vi "toplevel.vi"() -> ()   [LabVIEW 2013]
uses:
  SensorDataType.ctl
panel:
  out "Einfallswinkel":dbl(knob) scale=-90.0..90.0
  out "Sensordaten (Raw)":u16[](graph)
  in  "Simulated Orientation":i8(knob) scale=-90.0..90.0
  out "Simulation":bool
  out "Live-Daten":bool
  in  "Modus Operandi":bool
  out "Sensordaten (Normalisiert)":dbl[](graph)=[0.10526315789473684, 0.15789473684210525, 0.15789473684210525, 0.15789473684210525, 0.15789473684210525, 0.10526315789473684, 0.15789473684210525]
  in  "stop":bool
  in  "Serial Input":refnum<visa-resource-name>="COM6"
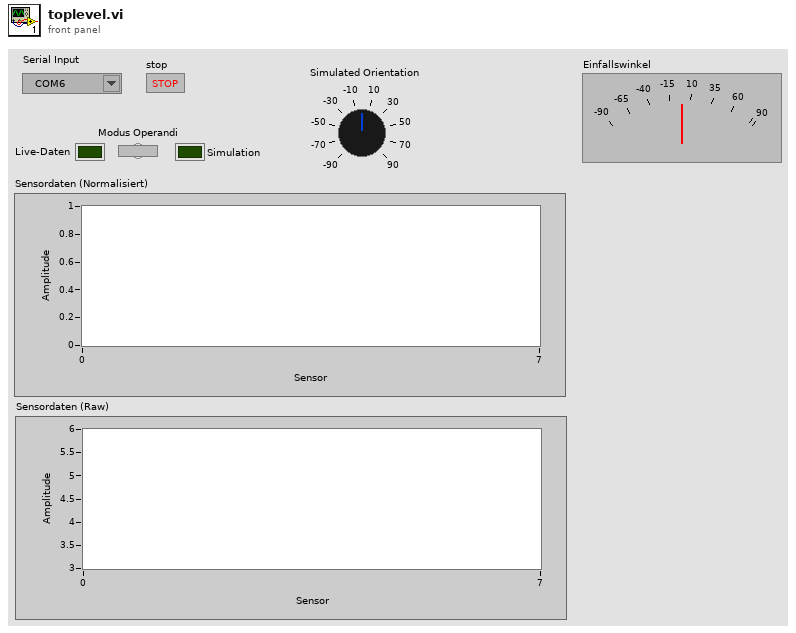
[diagram p1: front panel]
types:
  T1 = enum8{"Enabled", "Disabled", "Disabled and Grayed Out"}
  T2 = typedef "SensorDataType.ctl" = cluster{"Raw":u16[], "Normalized\n":dbl[]}
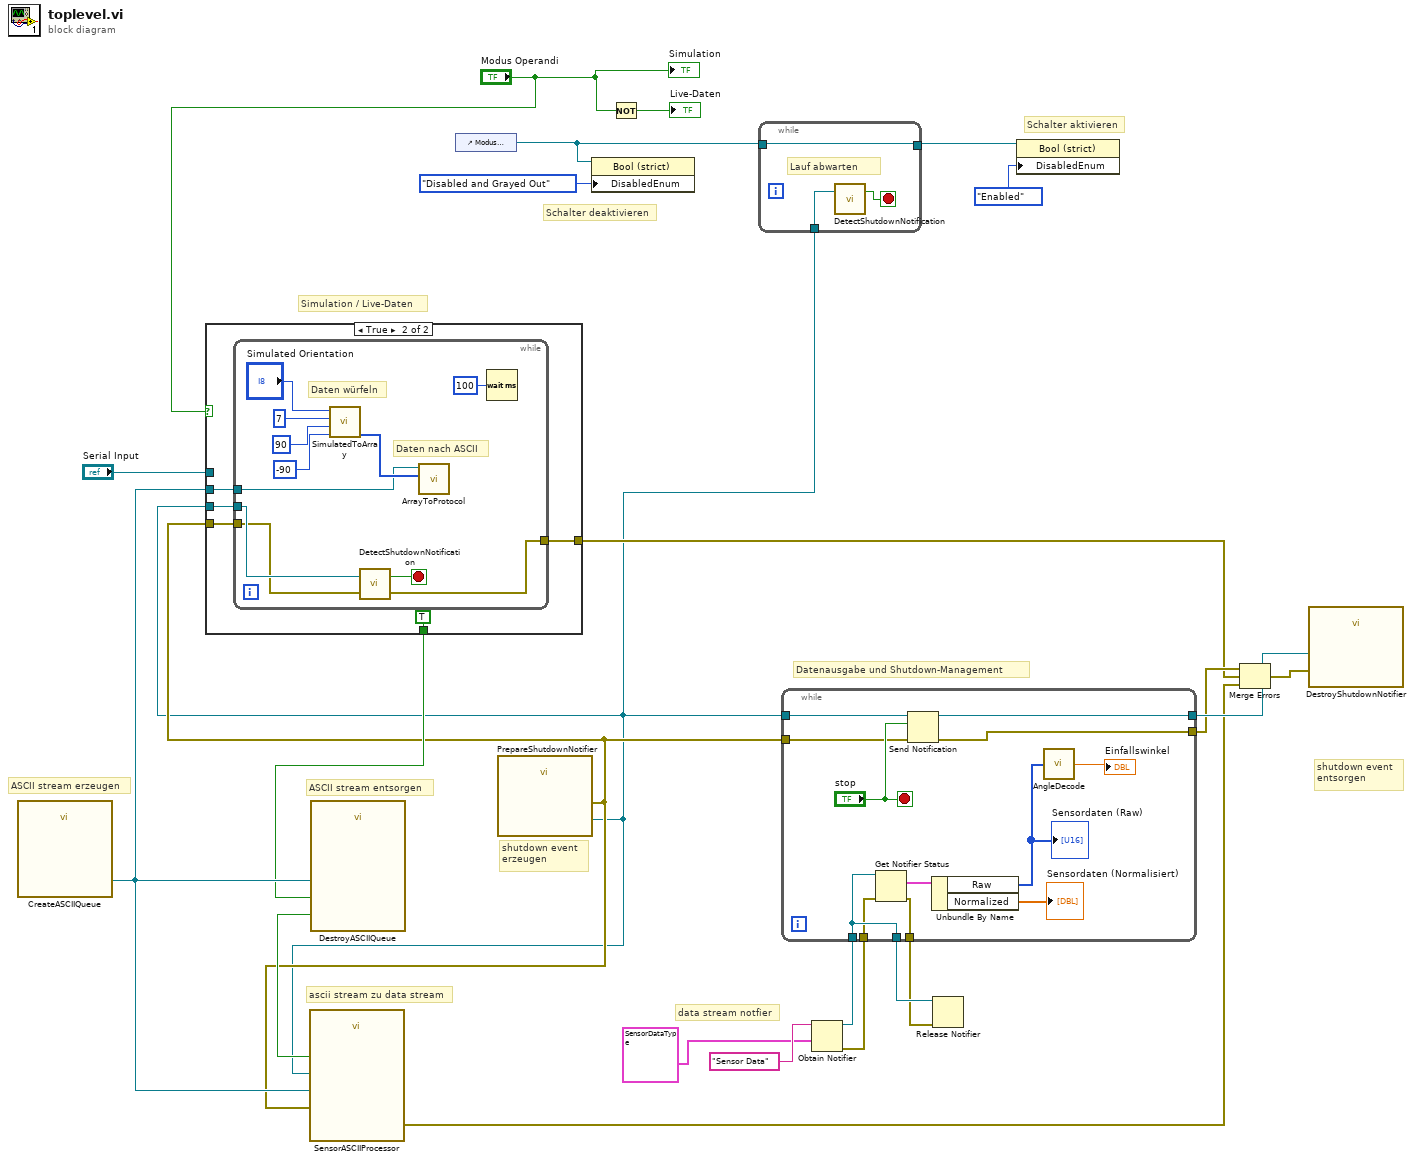
[diagram p0: block diagram]
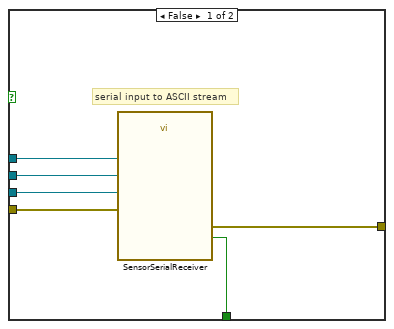
[diagram p2: hidden frame]
diagram:
  # "Simulation / Live-Daten"
  # "Schalter deaktivieren"
  # "Schalter aktivieren"
  # "Datenausgabe und Shutdown-Management"
  # "shutdown event\nentsorgen"
  # "data stream notfier"
  # "shutdown event\nerzeugen"
  # "ASCII stream entsorgen"
  # "ASCII stream erzeugen"
  # "ascii stream zu data stream"
  n1 = call "CreateASCIIQueue.vi"() -> ("Queue out"=w20:refnum<queue>)  [unwired: 11 in]
  n2 = control-ref of="Modus Operandi"() -> (w3:refnum<vi>)
  n3 = call "PrepareShutdownNotifier.vi"() -> ("error out"=w8:errorcluster, "Notifier out"=w7:refnum<notifier>)  [unwired: 10 in]
  n4 = case shown="True" "Modus Operandi" {
    tunnel: "Serial Input" -> [w29 _]
    tunnel: w20 -> [w28 w30]
    tunnel: [w27 w32] -> w19
    tunnel: [w26 TRUE ("Done")] -> w15
    tunnel: w8 -> [w25 w31]
    tunnel: w7 -> [w24 w34]
    frame False {
      # "serial input to ASCII stream"
      n5 = call "SensorSerialReceiver.vi"("Notifier Error In"=w25, "Notifier"=w24, "Queue"=w28, "VISA resource name"=w29) -> ("Notifier Error Out"=w27:errorcluster, "Done"=w26:bool)  [unwired: 6 in]
    }
    frame True {
      n6 = while {
        tunnel: w34 -> [w40]
        tunnel: [w39] -> w32
        tunnel: w31 -> [w38]
        tunnel: w30 -> [w36]
        stop <- w41 stop-if-true
        # "Daten nach ASCII"
        # "Daten würfeln"
        n7 = call "SimulatedToArray.vi"("Minimum Angle"=i8 -90, "Maximum Angle"=i8 90, "Number of Elements"=u8 7, "Degree"="Simulated Orientation") -> ("Value Array"=w37:u16[])  [unwired: 7 in]
        n8 = call "DetectShutdownNotification.vi"("error in (no error)"=w38, "Shutdown Notifier"=w40) -> ("error out"=w39:errorcluster, "Shutdown"=w41:bool)
        n9 = call "ArrayToProtocol.vi"("Simulated Data"=w37, "Queue"=w36) -> ()  [unwired: 10 in]
        n10 = Wait (ms)(milliseconds to wait=u32 100) -> ()  [unwired: 1 out]
      }
    }
  }
  n11 = call "SensorASCIIProcessor.vi"("Notifier Error In"=w8, "Shutdown Notifier"=w7, "Queue"=w20) -> ("Notifier Error Out"=w18:errorcluster, "Done"=w17:bool)  [unwired: 4 in]
  n12 = call "DestroyASCIIQueue.vi"("Ready 2"=w17, "Ready 1"=w15, "Queue in"=w20) -> ()  [unwired: 9 in]
  n13 = property on="Property Node" class="Bool (strict)"(reference=w3, "DisabledEnum"=T1."Disabled and Grayed Out" ("Disabled")) -> ()  [unwired: 1 in, 2 out]
  n14 = Not(x="Modus Operandi") -> (.not. x?=→"Live-Daten":bool)
  n15 = while {
    tunnel: w7 -> [w48]
    tunnel: [w46] -> w4
    tunnel: w3 -> [w46]
    stop <- w47 stop-if-true
    # "Lauf abwarten"
    n16 = call "DetectShutdownNotification.vi"("Shutdown Notifier"=w48) -> ("Shutdown"=w47:bool)  [unwired: 1 in, 1 out]
  }
  n17 = Obtain Notifier(name (unnamed)="Sensor Data", notification data type=T2 {"Raw"=[22, 22, 26, 24, 24, 26, 26], "Normalized\n"=[0.12941176470588237, 0.12941176470588237, 0.15294117647058825, 0.1411764705882353, 0.1411764705882353, 0.15294117647058825, 0.15294117647058825]} ("Sensor Data Type")) -> (notifier out=w14:refnum<notifier>, error out=w11:errorcluster)  [unwired: 2 in, 1 out]
  n18 = while {
    tunnel: w7 -> [w51]
    tunnel: [w59] -> w23
    tunnel: [w58] -> w22
    tunnel: w8 -> [w57]
    tunnel: w14 -> [w54]
    tunnel: [w54] -> w13
    tunnel: [w53] -> w12
    tunnel: w11 -> [w52]
    stop <- "stop" stop-if-true
    n19 = Get Notifier Status(notifier=w54, error in (no error)=w52) -> (current notification=w56:T2, error out=w53:errorcluster)  [unwired: 3 out]
    n20 = Send Notification(notification="stop", notifier=w51, error in (no error)=w57) -> (notifier out=w59:refnum<notifier>, error out=w58:errorcluster)
    n21 = Unbundle By Name(w56) -> ("Raw"=w50:u16[], "Normalized"=→"Sensordaten (Normalisiert)":dbl[])
    "Sensordaten (Raw)" <- w50
    n22 = call "AngleDecode.vi"("Data"=w50) -> ("Peak Angle"=→"Einfallswinkel":dbl)
  }
  n23 = Release Notifier(notifier=w13, error in (no error)=w12) -> ()  [unwired: 1 in, 3 out]
  n24 = property on="Property Node" class="Bool (strict)"(reference=w4, "DisabledEnum"=T1."Enabled" ("Disabled")) -> ()  [unwired: 1 in, 2 out]
  n25 = Merge Errors(w22, w19, w18) -> (w9:errorcluster)
  n26 = call "DestroyShutdownNotifier.vi"("error in (no error)"=w9, "Notifier in"=w23) -> ()  [unwired: 10 in]
  "Simulation" <- "Modus Operandi"
